vi "Assert Error Code.vi"(4 "Execution time (s)":dbl=-1.0, 5 "Assert Only? (F)":bool, 6 "error code (1)":i32=1, 7 "Assert specific error code":i32, 8 "error in (no error)":errorcluster, 11 "Error?":errorcluster) -> (0 "error out":errorcluster)   [LabVIEW 2019, in "Sports Unit Tests.lvclass"]
uses:
  Sports Unit Tests.lvclass
  <vilib>/addons/_JKI Toolkits/Caraya/classes/Assert/Assert Error.vi
  <vilib>/addons/_JKI Toolkits/Caraya/classes/Assert/Assert Equal Value_Variant.vi
  <vilib>/addons/_JKI Toolkits/Caraya/classes/Assert/Assert.lvclass
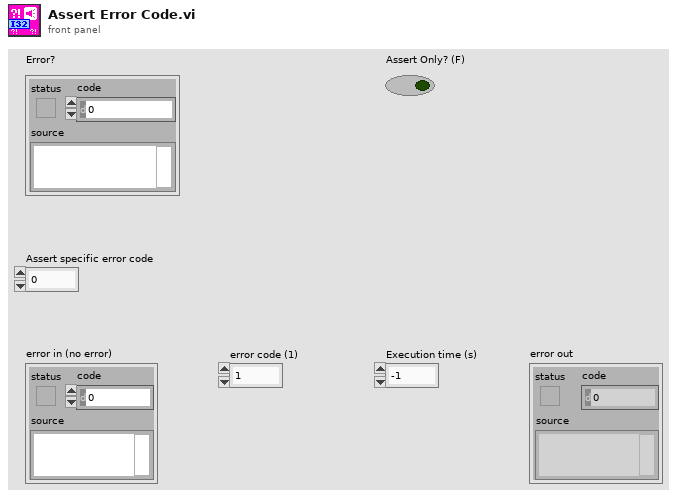
[diagram p1: front panel]
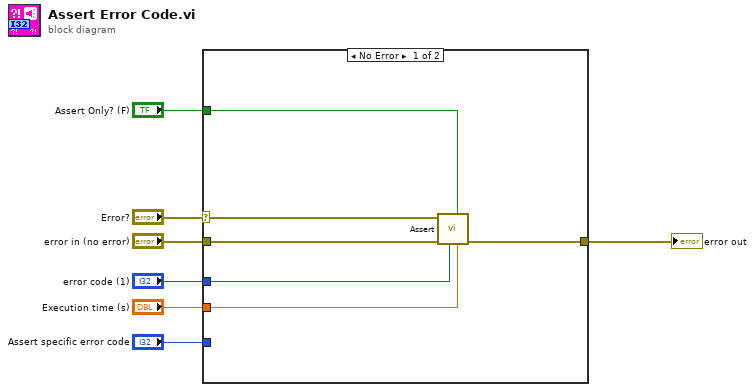
[diagram p0: block diagram]
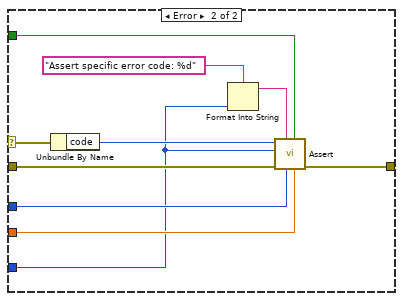
[diagram p2: hidden frame]
diagram:
  n1 = case shown="No Error" "Error?" {
    selector: "Error?" -> [w8 w23]
    tunnel: "error in (no error)" -> [w13 w21]
    tunnel: "Assert Only? (F)" -> [w12 w20]
    tunnel: "error code (1)" -> [w11 w19]
    tunnel: "Execution time (s)" -> [w10 w18]
    tunnel: [w9 w17] -> w3
    tunnel: "Assert specific error code" -> [_ w16]
    frame No Error {
      n2 = call-poly <vilib>:"Assert.vi"("Execution time (s)"=w10, "Assert Only? (F)"=w12, "error code (1)"=w11, "error in (no error)"=w13, "Error?"=w8) -> ("error out"=w9:errorcluster)  [unwired: 6 in]
    }
    frame Error {
      n3 = Unbundle By Name(w23) -> ("code"=w22:i32)
      n4 = Format Into String(format string="Assert specific error code: %d" ("Label"), w16) -> (resulting string=w14:string)  [unwired: 2 in, 1 out]
      n5 = call-poly <vilib>:"Assert.vi"("Execution time (s)"=w18, "Assert Only? (F)"=w20, "error code (1)"=w19, "Label"=w14, "error in (no error)"=w21, "Y"=w16, "X"=w22) -> ("error out"=w17:errorcluster)  [unwired: 4 in]
    }
  }
  "error out" <- w3
